vi "Current View.vi"() -> ()   [LabVIEW 2013]
uses:
  <vilib>/Instr/_visa.llb/VISA Configure Serial Port (Instr).vi
panel:
  out "VISA resource name out":refnum<visa-resource-name>
  in  "Tab Control":enum32{"CONTROLS", "GRAPH"}(tab)
  out "Yellow":dbl(graph)
  out "Red":dbl(graph)
  out "Blue":dbl(graph)
  in  "Stop button":bool
  in  "COM PORT":refnum<visa-resource-name>="COM3"
  out "YELLOW PHASE":dbl
  out "BLUE PHASE":dbl
  out "RED PHASE":dbl
  out "VOLTAGE UNBALANCE CALC(%)":dbl
  out "WAVE FORM GRAPH":dbl[][](graph)
  # "VOLTAGE UNBALANCE MONITORING"
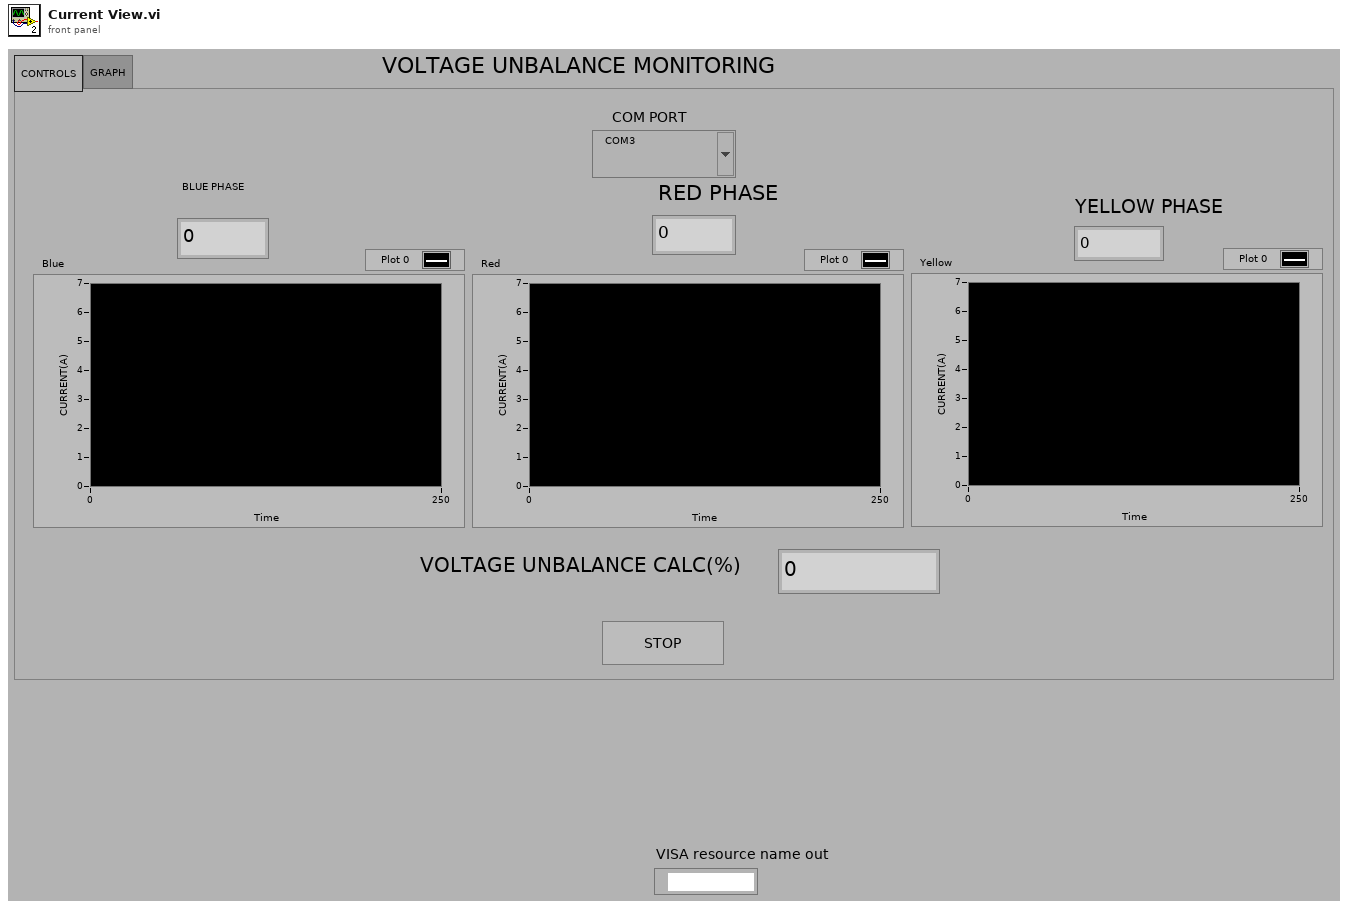
[diagram p1: front panel]
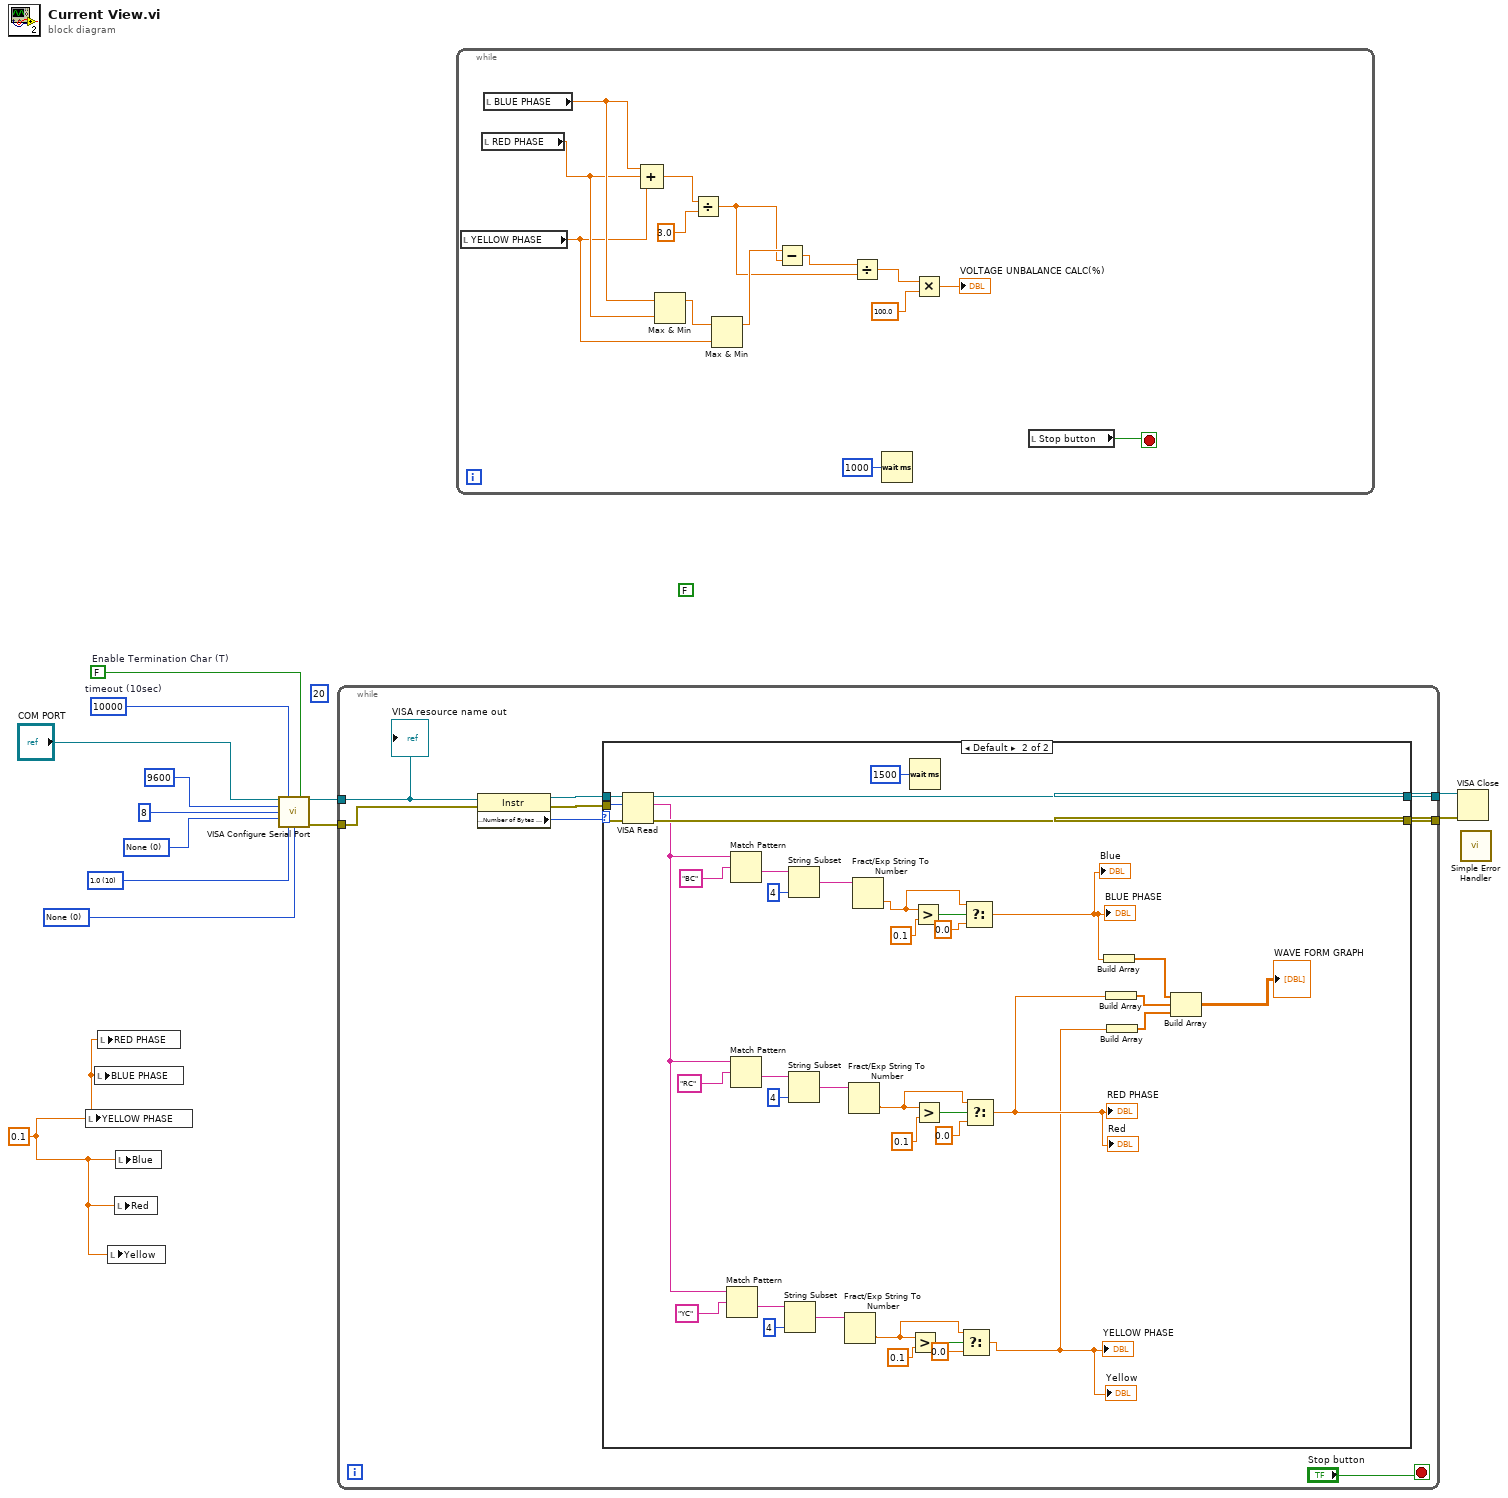
[diagram p0: block diagram]
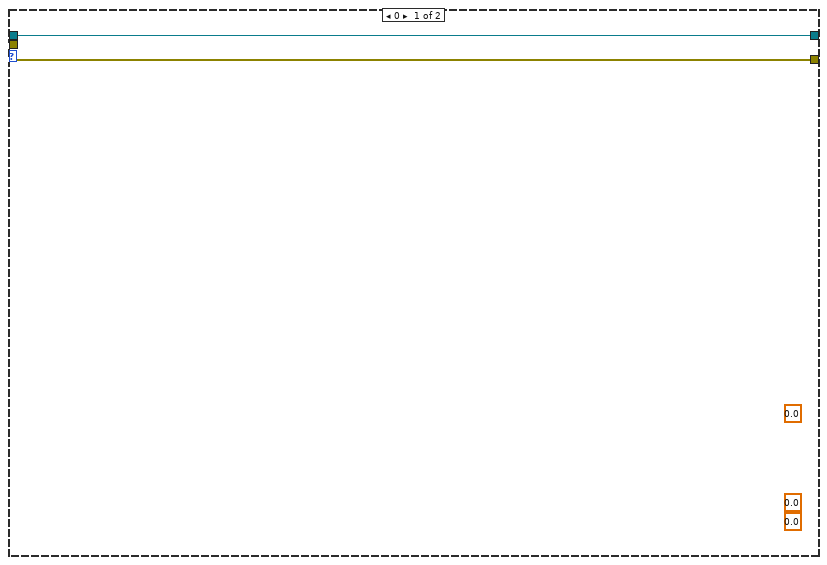
[diagram p2: hidden frame]
diagram:
  (unwired) 20
  w1 = 0.1 ("y")
  w8 = u16 0 items=["None"=0, "XON/XOFF"=1, "RTS/CTS"=2, "DTR/DSR"=4] ("flow control")
  w9 = u16 10 items=["1.0"=10, "1.5"=15, "2.0"=20] ("stop bits")
  w12 = u16 0 items=["None", "Odd", "Even", "Mark", "Space"] ("parity")
  w10 = FALSE  # Enable Termination Char (T)
  w11 = u32 10000  # timeout (10sec)
  (unwired) FALSE
  n1 = local write "YELLOW PHASE"(w1) -> ()
  n2 = local write "BLUE PHASE"(w1) -> ()
  n3 = local write "RED PHASE"(w1) -> ()
  n4 = local write "Yellow"(w1) -> ()
  n5 = local write "Red"(w1) -> ()
  n6 = local write "Blue"(w1) -> ()
  n7 = call-poly "VISA Configure Serial Port"("VISA resource name"="COM PORT", "timeout (10sec)"=w11, "Enable Termination\nChar (T)"=w10, "baud rate (9600)"=u32 9600 ("baud rate"), "data bits (8)"=u16 8 ("data bits"), "parity (0:none)"=w12, "stop bits (10: 1 bit)"=w9, "flow control (0:none)"=w8) -> ("VISA resource name out"=w5:refnum<visa-resource-name>, "error out"=w4:errorcluster)  [unwired: 1 in, 5 out]
  n8 = while {
    tunnel: w5 -> [w14]
    tunnel: w4 -> [w16]
    tunnel: [w18] -> w3
    tunnel: [w17] -> w2
    stop <- "Stop button" stop-if-true
    n9 = property class="Instr"(reference=w14, error in=w16) -> (reference out=w21:refnum<visa-resource-name>, error out=w20:errorcluster, "Serial Settings:Number of Bytes at Serial Port"=w19:u32)
    n10 = case shown="Default" w19 {
      selector: w19 -> [_ w59]
      tunnel: w21 -> [w22 w61]
      tunnel: w20 -> [w23 w60]
      tunnel: [w23 w58] -> w17
      tunnel: [w22 w57] -> w18
      frame 0 {
        (unwired) 0.0 ("f")
        (unwired) 0.0 ("f")
        (unwired) 0.0 ("f")
      }
      frame Default {
        n11 = VISA Read(VISA resource name=w61, byte count=w59, error in (no error)=w60) -> (VISA resource name out=w57:refnum<visa-resource-name>, read buffer=w31:string, error out=w58:errorcluster)  [unwired: 1 out]
        n12 = Match Pattern(string=w31, regular expression="YC") -> (after substring=w33:string)  [unwired: 1 in, 3 out]
        n13 = Match Pattern(string=w31, regular expression="BC") -> (after substring=w55:string)  [unwired: 1 in, 3 out]
        n14 = Match Pattern(string=w31, regular expression="RC") -> (after substring=w52:string)  [unwired: 1 in, 3 out]
        n15 = String Subset(string=w33, length (rest)=4 ("length (rest)")) -> (substring=w35:string)  [unwired: 1 in]
        n16 = String Subset(string=w55, length (rest)=4 ("length (rest)")) -> (substring=w50:string)  [unwired: 1 in]
        n17 = String Subset(string=w52, length (rest)=4 ("length (rest)")) -> (substring=w49:string)  [unwired: 1 in]
        n18 = Fract/Exp String To Number(string=w35) -> (number=w38:dbl)  [unwired: 3 in, 1 out]
        n19 = Fract/Exp String To Number(string=w49) -> (number=w42:dbl)  [unwired: 3 in, 1 out]
        n20 = Fract/Exp String To Number(string=w50) -> (number=w43:dbl)  [unwired: 3 in, 1 out]
        n21 = Wait (ms)(milliseconds to wait=u32 1500) -> ()  [unwired: 1 out]
        n22 = Greater?(x=w38, y=0.1) -> (0:w37:bool)
        n23 = Greater?(x=w43, y=0.1) -> (0:w44:bool)
        n24 = Greater?(x=w42, y=0.1) -> (0:w45:bool)
        n25 = Select(t=w38, s=w37, f=0.0) -> (s? t:f=w28:dbl)
        "YELLOW PHASE" <- w28
        "Yellow" <- w28
        n26 = Select(t=w43, s=w44, f=0.0) -> (s? t:f=w30:dbl)
        "BLUE PHASE" <- w30
        "Blue" <- w30
        n27 = Select(t=w42, s=w45, f=0.0) -> (s? t:f=w29:dbl)
        "RED PHASE" <- w29
        "Red" <- w29
        n28 = Build Array(w30) -> (w27:dbl[])
        n29 = Build Array(w29) -> (w26:dbl[])
        n30 = Build Array(w28) -> (w25:dbl[])
        n31 = Build Array(w27, w26, w25) -> (→"WAVE FORM GRAPH":dbl[][])
      }
    }
    "VISA resource name out" <- w14
  }
  n32 = while {
    stop <- w75 stop-if-true
    n33 = local read "YELLOW PHASE"() -> (w68:dbl)
    n34 = local read "RED PHASE"() -> (w70:dbl)
    n35 = local read "BLUE PHASE"() -> (w71:dbl)
    n36 = Compound Arithmetic op=ADD(w71, w70, w68) -> (w73:dbl)
    n37 = Max & Min(x=w71, y=w70) -> (max(x,y)=w69:dbl)  [unwired: 1 out]
    n38 = Divide(x=w73, y=3.0) -> (x/y=w65:dbl)
    n39 = Max & Min(x=w69, y=w68) -> (max(x,y)=w67:dbl)  [unwired: 1 out]
    n40 = Subtract(x=w67, y=w65) -> (x-y=w66:dbl)
    n41 = Divide(x=w66, y=w65) -> (x/y=w64:dbl)
    n42 = Wait (ms)(milliseconds to wait=u32 1000) -> ()  [unwired: 1 out]
    n43 = Multiply(x=w64, y=100.0) -> (x*y=→"VOLTAGE UNBALANCE CALC(%)":dbl)
    n44 = local read "Stop button"() -> (w75:bool)
  }
  n45 = VISA Close(VISA resource name=w3, error in (no error)=w2) -> ()  [unwired: 1 out]
  n46 = call <vilib>:"Simple Error Handler.vi"() -> ()  [unwired: 2 in, 8 out]
